vi "Empty Buffer.vi"(8 "error in (no error)":errorcluster, 11 "OXY_SCPI Reseource In":refnum<visa-resource-name>) -> (0 "error out":errorcluster, 3 "OXY_SCPI Reseource Out":refnum<visa-resource-name>)   [LabVIEW 2020, in "OXYGEN_Datastream.lvlib"]
uses:
  OXYGEN_Datastream.lvlib
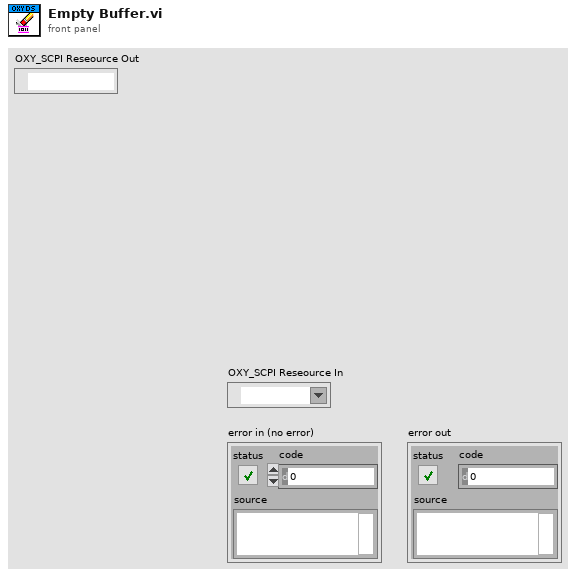
[diagram p1: front panel]
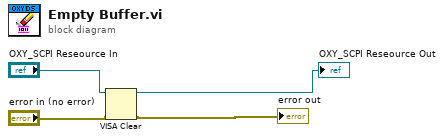
[diagram p0: block diagram]
diagram:
  n1 = VISA Clear(VISA resource name="OXY_SCPI Reseource In", error in (no error)="error in (no error)") -> (VISA resource name out=→"OXY_SCPI Reseource Out":refnum<visa-resource-name>, error out=→"error out":errorcluster)
